vi "字符键盘.vi"(10 "显示样式":u32, 11 "原值":string) -> (3 "x+y":string)   [LabVIEW 2016, in "数据传输系统.lvlib"]
uses:
  <vilib>/event_ctls.llb/eventvkey.ctl
panel:
  in  "M":bool
  in  "N":bool
  in  "B":bool
  in  "V":bool
  in  "C":bool
  in  "X":bool
  in  "Z":bool
  in  "L":bool
  in  "K":bool
  in  "J":bool
  in  "H":bool
  in  "G":bool
  in  "F":bool
  in  "D":bool
  in  "S":bool
  in  "A":bool
  in  "P":bool
  in  "O":bool
  in  "I":bool
  in  "U":bool
  in  "Y":bool
  in  "T":bool
  in  "R":bool
  in  "E":bool
  in  "W":bool
  in  "Q":bool
  in  "清除":bool
  in  "退格":bool
  in  "取消按钮":bool
  in  "_":bool
  out "字符串":string
  in  "0":bool
  in  "停止":bool
  in  "9":bool
  in  "8":bool
  in  "7":bool
  in  "6":bool
  in  "5":bool
  in  "4":bool
  in  "3":bool
  in  "2":bool
  in  "1":bool
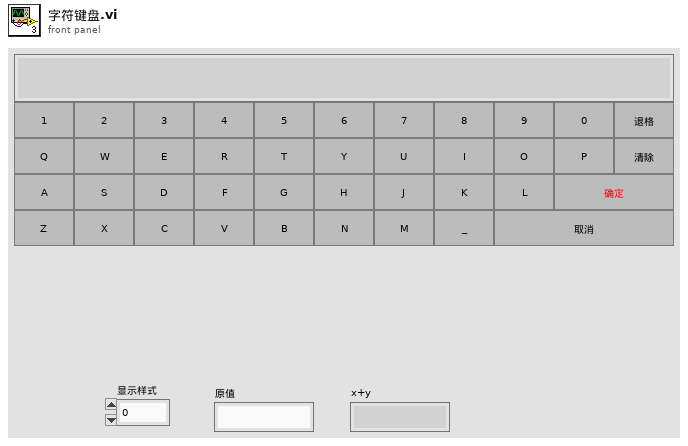
[diagram p1: front panel]
types:
  T1 = typedef "eventvkey.ctl" = enum16{"ASCII", "Enter", "Return", "Shift", "Ctrl", "Alt", "Cmd", "Opt", "Caps", "NumLock", "Clear", "Break", "Up", "Down", "Left", "Right", "Insert", "Delete", "Home", "End", "PageUp", "PageDown", "Escape", "Help", "Pause", "ScrollLock", "F1", "F2", "F3", "F4", "F5", "F6", "F7", "F8", "F9", "F10", "F11", "F12", "F13", "F14", "F15", "F16", "F17", "F18", "F19", "F20", "F21", "F22", "F23", "F24", "Play", "VolumeUp", "VolumeDown", "Mute", "Two Byte Char"}
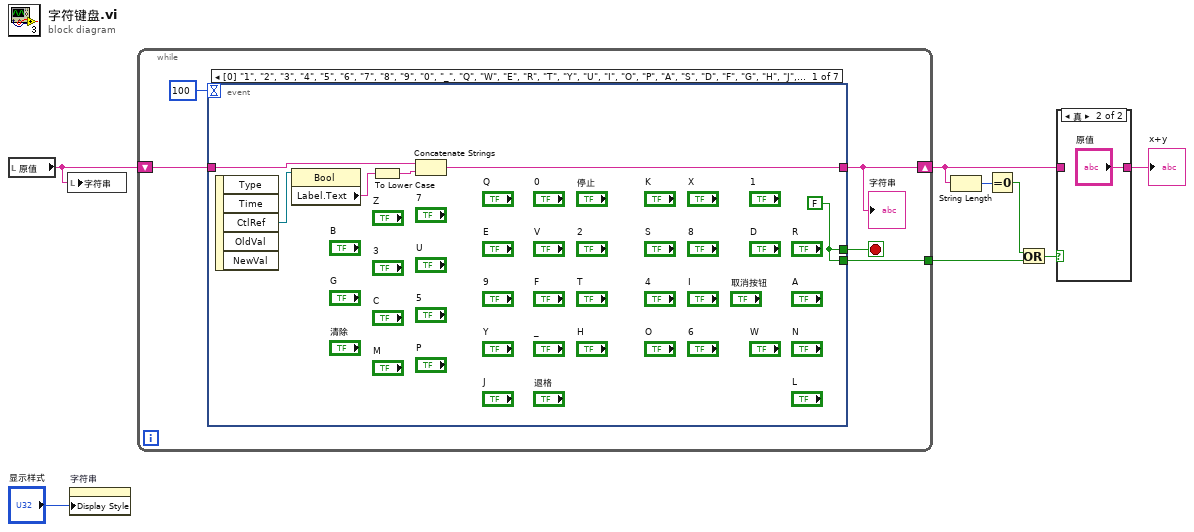
[diagram p0: block diagram]
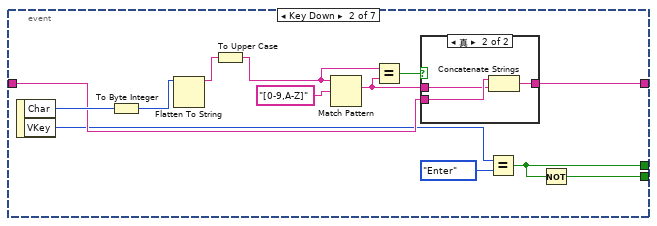
[diagram p3: hidden frame]
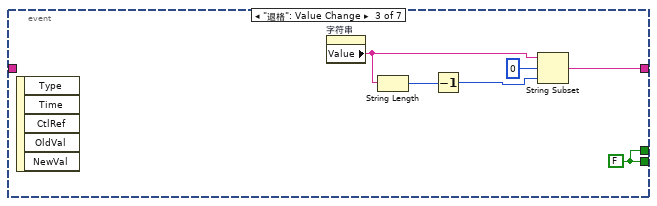
[diagram p5: hidden frame]
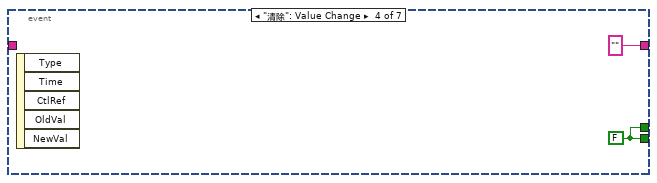
[diagram p6: hidden frame]
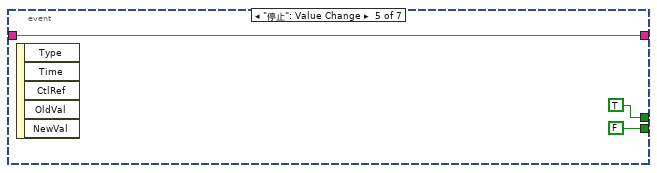
[diagram p7: hidden frame]
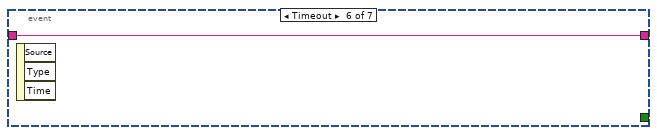
[diagram p8: hidden frame]
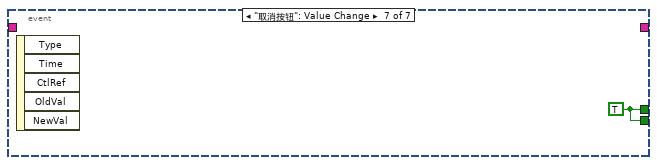
[diagram p9: hidden frame]
diagram:
  n1 = local read "原值"() -> (w1:string)
  n2 = local write "字符串"(w1) -> ()
  n3 = property on="字符串" class="Str"("Display Style"="显示样式") -> ()  [unwired: 2 in, 2 out]
  n4 = while {
    shift-right: [w12] -> w8
    shift-left: w1 -> [w11]
    tunnel: [w10] -> w3
    stop <- w13 stop-if-true
    n5 = event shown="[0] \"1\", \"2\", \"3\", \"4\", \"5\", \"6\", \"7\", \"8\", \"9\", \"0\", \"_\", \"Q\", \"W\", \"E\", \"R\", \"T\", \"Y\", \"U\", \"I\", \"O\", \"P\", \"A\", \"S\", \"D\", \"F\", \"G\", \"H\", \"J\", \"K\", \"L\", \"Z\", \"X\", \"C\", \"V\", \"B\", \"N\", \"M\": 值改变" {
      selector: _ -> [_ _ _ _ _ _ _]
      dyn-events: _ -> [_ _ _ _ _ _ _]
      timeout: 100 -> [_ _ _ _ _ _ _]
      tunnel: [w16 w23 w37 w43 TRUE _ w49] -> w13
      tunnel: [w18 w30 w38 "" ("Label.Text") w46 w48 _] -> w12
      tunnel: w11 -> [w17 w29 _ _ w46 w48 _]
      tunnel: [w16 w24 w37 w43 FALSE _ w49] -> w10
      event "1", "2", "3", "4", "5", "6", "7", "8", "9", "0", "_", "Q", "W", "E", "R", "T", "Y", "U", "I", "O", "P", "A", "S", "D", "F", "G", "H", "J", "K", "L", "Z", "X", "C", "V", "B", "N", "M": Value Change {
        w16 = FALSE
        n6 = event-data() -> ("CtlRef"=w19:refnum<vi>)  [unwired: 1 in, 4 out]
        n7 = property class="Bool"(reference=w19) -> ("Label.Text"=w14:string)  [unwired: 1 in, 2 out]
        n8 = To Lower Case(string=w14) -> (all lower case string=w15:string)
        n9 = Concatenate Strings(w17, w15) -> (w18:string)
      }
      event Key Down {
        n10 = event-data() -> ("Char"=w32:i16, "VKey"=w22:T1)  [unwired: 1 in]
        n11 = To Byte Integer(number=w32) -> (8bit integer=w31:i8)
        n12 = Flatten To String(anything=w31) -> (data string=w21:string)  [unwired: 3 in, 2 out]
        n13 = To Upper Case(1:w21) -> (0:w20:string)
        n14 = Match Pattern(string=w20, regular expression="[0-9,A-Z]" ("正则表达式")) -> (match substring=w27:string)  [unwired: 1 in, 3 out]
        n15 = Equal?(x=w20, y=w27) -> (x = y?=w26:bool)
        n16 = case shown="真" w26 {
          tunnel: [w33 w36] -> w30
          tunnel: w29 -> [w33 w35]
          tunnel: w27 -> [_ w34]
          frame False {
          }
          frame True {
            n17 = Concatenate Strings(w35, w34) -> (w36:string)
          }
        }
        n18 = Equal?(x=w22, y=eventvkey."Enter" ("V键")) -> (x = y?=w23:bool)
        n19 = Not(x=w23) -> (.not. x?=w24:bool)
      }
      event "退格": Value Change {
        w37 = FALSE
        n20 = event-data() -> ()  [unwired: 1 in, 5 out]
        n21 = property on="字符串" class="Str"() -> ("Value"=w41:string)  [unwired: 2 in, 2 out]
        n22 = String Length(string=w41) -> (length=w42:i32)
        n23 = Decrement(x=w42) -> (x-1=w39:i32)
        n24 = String Subset(string=w41, offset (0)=0 ("偏移量(0)"), length (rest)=w39) -> (substring=w38:string)
      }
      event "清除": Value Change {
        w43 = FALSE
        n25 = event-data() -> ()  [unwired: 1 in, 5 out]
      }
      event "停止": Value Change {
        n26 = event-data() -> ()  [unwired: 1 in, 5 out]
      }
      event Timeout {
        n27 = event-data() -> ()  [unwired: 1 in, 3 out]
      }
      event "取消按钮": Value Change {
        w49 = TRUE
        n28 = event-data() -> ()  [unwired: 1 in, 5 out]
      }
    }
    "字符串" <- w12
  }
  n29 = String Length(string=w8) -> (length=w7:i32)
  n30 = Equal To 0?(x=w7) -> (x = 0?=w6:bool)
  n31 = Or(x=w6, y=w3) -> (x .or. y?=w5:bool)
  n32 = case shown="真" w5 {
    tunnel: w8 -> [w50 _]
    tunnel: [w50 "原值"] -> w4
    frame False {
    }
    frame True {
    }
  }
  "x+y" <- w4
